vi "Undo.vi"(0 "reference in":refnum<class "StopMusicCommand.lvclass">, 11 "Error In":errorcluster) -> (4 "reference out":refnum<class "StopMusicCommand.lvclass">, 15 "Error Out":errorcluster)   [LabVIEW 2024, in "StopMusicCommand.lvclass"]
doc: "Calls MediaPlayer and plays music (opposite of play)."
uses:
  StopMusicCommand.lvclass
  StopMusicCommand.lvclass/StopMusicCommand.ctl
  Receiver/MediaPlayer_class/MediaPlayer.lvclass
panel:
  # "Connector Pane"
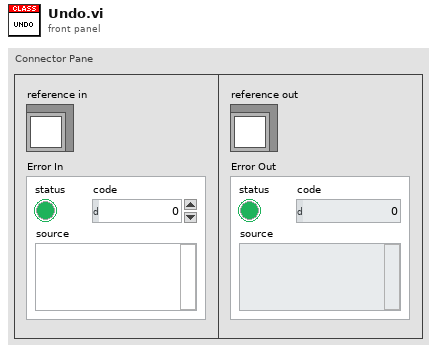
[diagram p1: front panel]
types:
  T1 = typedef "StopMusicCommand.lvclass/ObjectAttributes.ctl" = cluster{"MediaPlayerRef":refnum<class "MediaPlayer.lvclass">}
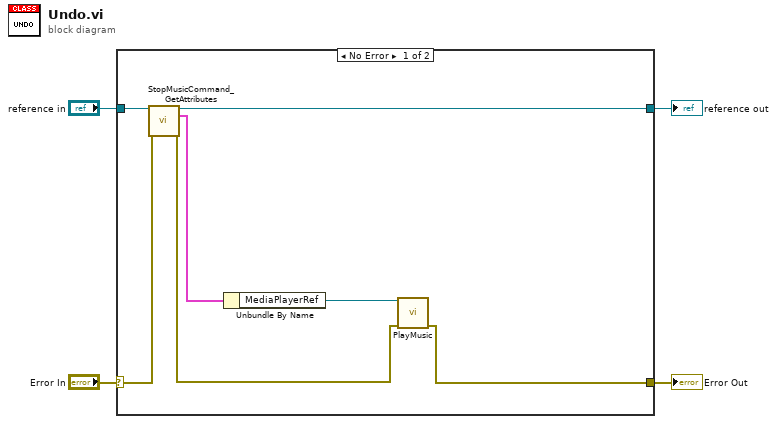
[diagram p0: block diagram]
diagram:
  n1 = case shown="No Error" "Error In" {
    selector: "Error In" -> [w11 w13]
    tunnel: [w6 w13] -> w3
    tunnel: [w7 w12] -> w1
    tunnel: "reference in" -> [w8 w12]
    frame No Error {
      n2 = call "StopMusicCommand_GetAttributes.vi"("reference in"=w8, "Error In"=w11) -> ("reference out"=w7:refnum<class "StopMusicCommand.lvclass">, "Data"=w10:T1, "Error Out"=w9:errorcluster)  [unwired: 10 in, 1 out]
      n3 = Unbundle By Name(w10) -> ("MediaPlayerRef"=w5:refnum<class "MediaPlayer.lvclass">)
      n4 = call-dynamic "PlayMusic.vi"("reference in"=w5, "Error In"=w9) -> ("Error Out"=w6:errorcluster)  [unwired: 11 in, 2 out]
    }
    frame Error {
    }
  }
  "Error Out" <- w3
  "reference out" <- w1
